vi "Instrument Manager Loop.vi"(8 "System Control":refnum<queue>, 11 "Instrument Manager":refnum<queue>) -> (0 "error out":errorcluster)   [LabVIEW 2020, in "ChromTech Series III Plugin.lvlib" / "Instrument Manager.lvlib"]
uses:
  Instrument Manager/Instrument Manager.lvlib
  support/Message Queue/Message Cluster.ctl
  Instrument Manager/Instrument State.ctl
  <vilib>/Utility/error.llb/Error Cluster From Error Code.vi
  <vilib>/ErrorRing/Error Ring.xnode
  support/Message Queue/Message Queue.lvlib
  ChromTech Series III Plugin.lvlib
  <instrlib>/ChromTech Series III Pump/ChromTech Series III Pump.lvlib
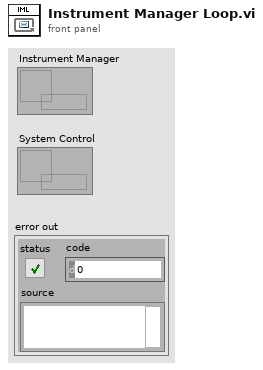
[diagram p1: front panel]
types:
  T1 = typedef "ChromTech Series III Plugin.lvlib/Instrument Manager.lvlib/Instrument State.ctl" = cluster{"VISA Resource":refnum<visa-resource-name>, "Flow Rate":dbl, "Running":bool, "Running Since":timestamp, "Pressure Data Point":cluster{"Time Stamp":timestamp, "Value":dbl}, "Upper Pressure Fault":bool, "Lower Pressure Fault":bool, "Motor Stall Fault":bool, "Sampling Rate (sec/sample)":dbl, "Retry Attempts":i32}
  T2 = cluster{"seconds since 1Jan1904":timestamp, "Pressure":i32}
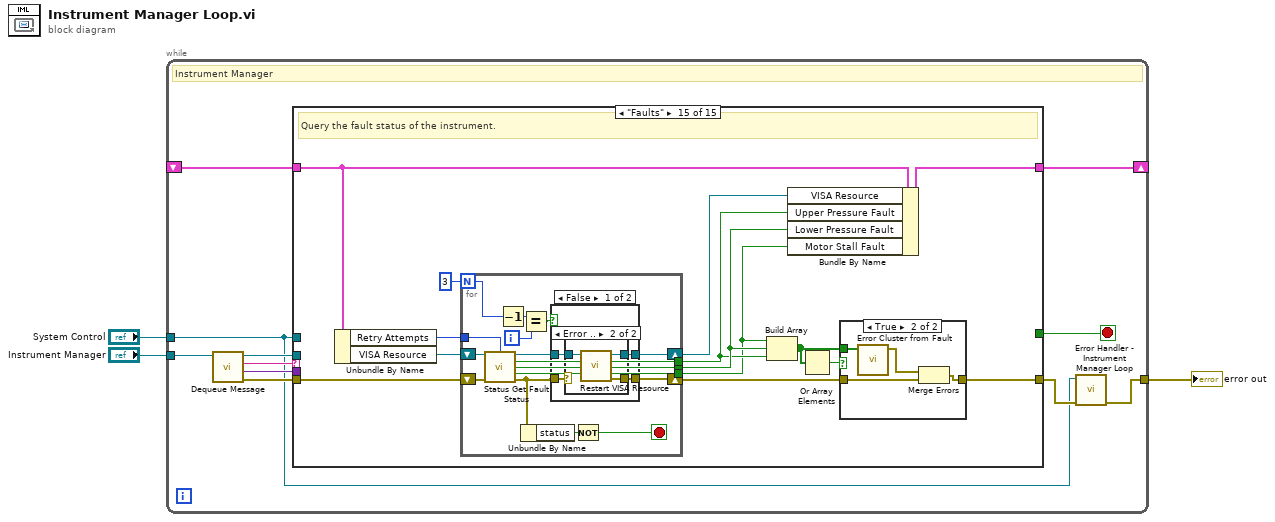
[diagram p0: block diagram]
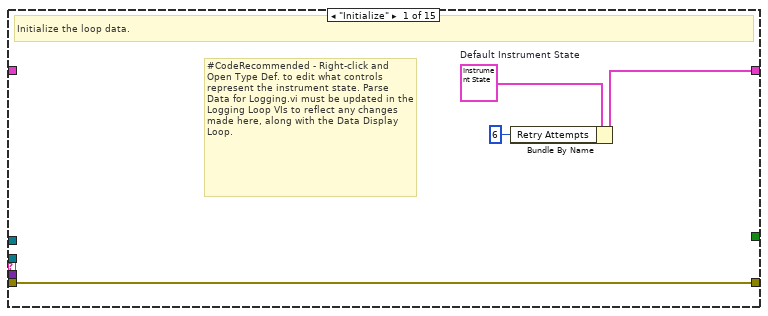
[diagram p2: hidden frame]
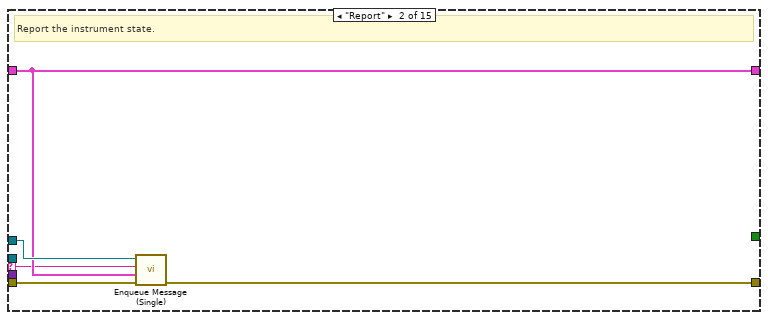
[diagram p3: hidden frame]
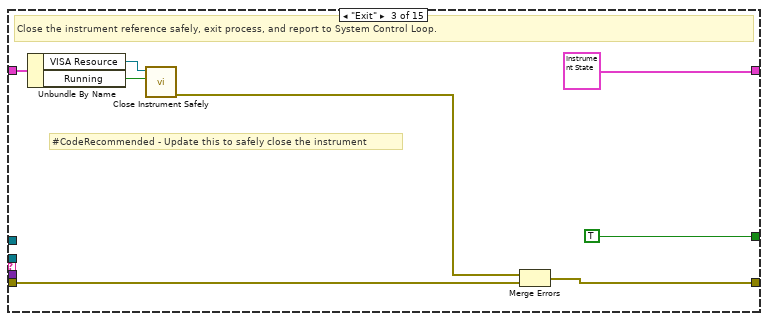
[diagram p4: hidden frame]
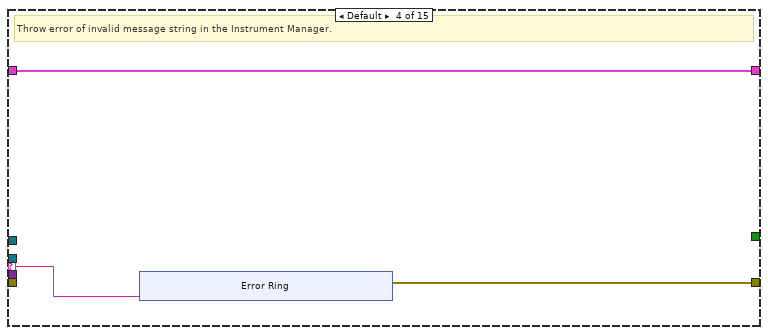
[diagram p5: hidden frame]
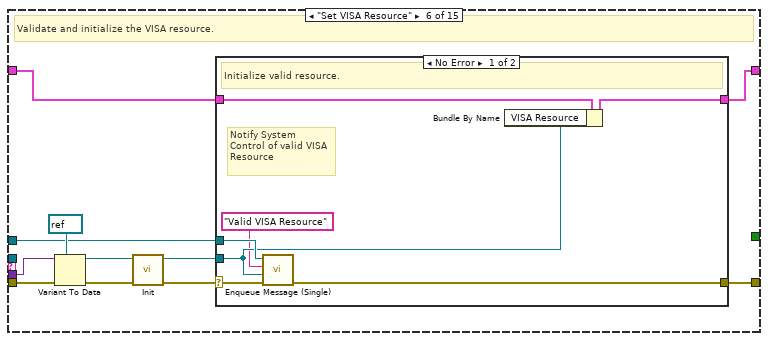
[diagram p7: hidden frame]
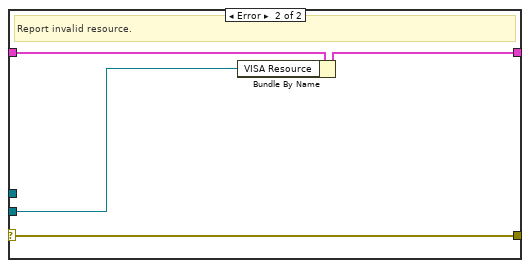
[diagram p8: hidden frame]
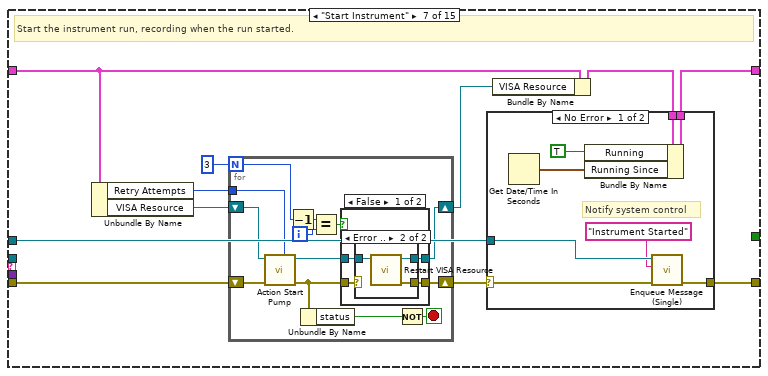
[diagram p9: hidden frame]
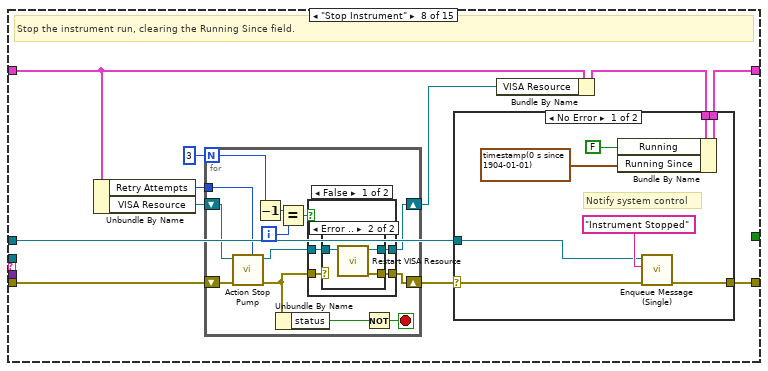
[diagram p13: hidden frame]
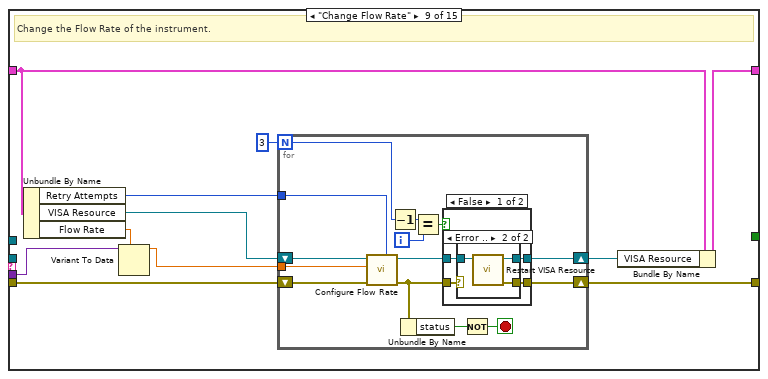
[diagram p17: hidden frame]
diagram:
  n1 = while {
    tunnel: "Instrument Manager" -> [w14]
    tunnel: "System Control" -> [w4]
    tunnel: [w8] -> w1
    shift-right: [w6] -> _
    shift-left: _ -> [w7]
    stop <- w5 stop-if-true
    # "Instrument Manager"
    n2 = call "Dequeue Message.vi"("Message Queue"=w14) -> ("error out"=w10:errorcluster, "Message Data"=w11:variant, "Message"=w13:string, "dup Message Queue"=w12:refnum<queue>)  [unwired: 7 in]
    n3 = case shown="\"Faults\"" w13 {
      selector: w13 -> [_ w19 _ w33 _ _ _ _ _ _ _ _ _ _ _]
      tunnel: w12 -> [_ _ _ _ _ _ _ _ _ _ _ _ _ _ _]
      tunnel: w4 -> [_ w22 _ _ _ w44 w75 w120 _ _ _ _ _ _ _]
      tunnel: w11 -> [_ _ _ _ _ w51 _ _ w166 _ w194 _ _ _ _]
      tunnel: w10 -> [w17 w23 w26 _ w42 w50 w73 w118 w161 w193 w199 w207 w240 w278 w317]
      tunnel: [w17 w21 w25 w32 w42 w54 w76 w121 w160 w193 w199 w206 w239 w276 w310] -> w9
      tunnel: w7 -> [_ w20 w31 w34 w43 w53 w72 w116 w165 w192 w196 w205 w241 w275 w314]
      tunnel: [w16 w20 T1 {"VISA Resource"="", "Flow Rate"=0.0, "Running"=FALSE, "Running Since"=timestamp(0 s since 1904-01-01), "Pressure Data Point"={"Time Stamp"=timestamp(0 s since 1904-01-01), "Value"=0.0}, "Upper Pressure Fault"=FALSE, "Lower Pressure Fault"=FALSE, "Motor Stall Fault"=FALSE, "Sampling Rate (sec/sample)"=0.0, "Retry Attempts"=0} w34 w43 w52 w74 w119 w157 w192 w195 w208 w244 w277 w316] -> w6
      tunnel: [_ _ TRUE _ _ _ _ _ _ _ _ _ _ _ _] -> w5
      frame "Initialize" {
        w18 = T1 {"VISA Resource"="", "Flow Rate"=0.0, "Running"=FALSE, "Running Since"=timestamp(0 s since 1904-01-01), "Pressure Data Point"={"Time Stamp"=timestamp(0 s since 1904-01-01), "Value"=0.0}, "Upper Pressure Fault"=FALSE, "Lower Pressure Fault"=FALSE, "Motor Stall Fault"=FALSE, "Sampling Rate (sec/sample)"=0.0, "Retry Attempts"=0}  # Default Instrument State
        # "#CodeRecommended - Right-click and Open Type Def. to edit what controls represent the instrument state. Parse Data for Logging.vi must be updated in the Logging Loop VIs to reflect any changes made here, along with the Data Display Loop."
        # "Initialize the loop data."
        n4 = Bundle By Name(cluster=w18, "Retry Attempts"=6) -> (w16:T1)
      }
      frame "Report" {
        # "Report the instrument state."
        n5 = call "Enqueue Message (Single).vi"("error in (no error)"=w23, "Message Data"=w20, "Message"=w19, "Message Queue"=w22) -> ("error out"=w21:errorcluster)  [unwired: 6 in, 1 out]
      }
      frame "Exit" {
        # "#CodeRecommended - Update this to safely close the instrument"
        # "Close the instrument reference safely, exit process, and report to System Control Loop."
        n6 = Unbundle By Name(w31) -> ("VISA Resource"=w29:refnum<visa-resource-name>, "Running"=w30:bool)
        n7 = call "Close Instrument Safely.vi"("Running (F)"=w30, "VISA Refnum in"=w29) -> ("error out"=w24:errorcluster)  [unwired: 9 in]
        n8 = Merge Errors(w24, w26) -> (w25:errorcluster)
      }
      frame Default {
        # "Throw error of invalid message string in the Instrument Manager."
        n9 = xnode "Error Ring"("parameter 0"=w33) -> ("error out"=w32:errorcluster)
      }
      frame "--- Copy This Frame ---" {
        # "Copy this frame and add responses to instrument specific messages."
      }
      frame "Set VISA Resource" {
        # "Validate and initialize the VISA resource."
        n10 = Variant To Data(error in=w50, type=refnum<visa-resource-name> refnum, Variant=w51) -> (data=w48:refnum<visa-resource-name>, error out=w49:errorcluster)
        n11 = call "Init.vi"("error in (no error)"=w49, "VISA resource in"=w48) -> ("error out"=w45:errorcluster, "VISA resource out"=w46:refnum<visa-resource-name>)  [unwired: 8 in]
        n12 = case shown="No Error" w45 {
          selector: w45 -> [w60 w62]
          tunnel: w46 -> [w57 w63]
          tunnel: [w59 w62] -> w54
          tunnel: w53 -> [w61 w65]
          tunnel: [w55 w64] -> w52
          tunnel: w44 -> [w58 _]
          frame No Error {
            # "Notify System Control of valid VISA Resource"
            # "Initialize valid resource."
            n13 = call "Enqueue Message (Single).vi"("error in (no error)"=w60, "Message Data"=w57, "Message"="Valid VISA Resource", "Message Queue"=w58) -> ("error out"=w59:errorcluster)  [unwired: 6 in, 1 out]
            n14 = Bundle By Name(cluster=w61, "VISA Resource"=w57) -> (w55:T1)
          }
          frame Error {
            # "Report invalid resource."
            n15 = Bundle By Name(cluster=w65, "VISA Resource"=w63) -> (w64:T1)
          }
        }
      }
      frame "Start Instrument" {
        # "Start the instrument run, recording when the run started."
        n16 = Unbundle By Name(w72) -> ("Retry Attempts"=w69:i32, "VISA Resource"=w71:refnum<visa-resource-name>)
        n17 = for {
          N: 3 -> [w80]
          tunnel: w69 -> [w88]
          shift-right: [w85] -> w70
          shift-left: w73 -> [w82]
          shift-right: [w77] -> w66
          shift-left: w71 -> [w89]
          i -> [w81]
          stop <- w86 stop-if-true
          n18 = call <instrlib>:"Action Start Pump.vi"("Retry Attempts (0)"=w88, "error in"=w82, "VISA resource name"=w89) -> ("error out"=w83:errorcluster, "VISA resource name out"=w84:refnum<visa-resource-name>)  [unwired: 7 in]
          n19 = Decrement(x=w80) -> (x-1=w79:i32)
          n20 = Unbundle By Name(w83) -> ("status"=w87:bool)
          n21 = Equal?(x=w79, y=w81) -> (x = y?=w78:bool)
          n22 = case shown="False" w78 {
            tunnel: [w93 w100] -> w85
            tunnel: w84 -> [w92 w99]
            tunnel: w83 -> [w91 w100]
            tunnel: [w90 w99] -> w77
            frame False {
              n23 = case shown="Error .." w91 {
                selector: w91 -> [w95 _]
                tunnel: [w95 w98] -> w93
                tunnel: w92 -> [w94 w97]
                tunnel: [w94 w96] -> w90
                frame No Error {
                }
                frame Error {
                  n24 = call "Restart VISA Resource.vi"("VISA Refnum in"=w97) -> ("error out"=w98:errorcluster, "VISA resource name out"=w96:refnum<visa-resource-name>)  [unwired: 9 in]
                }
              }
            }
            frame True {
            }
          }
          n25 = Not(x=w87) -> (.not. x?=w86:bool)
        }
        n26 = Bundle By Name(cluster=w72, "VISA Resource"=w66) -> (w67:T1)
        n27 = case shown="No Error" w70 {
          selector: w70 -> [w101 w110]
          tunnel: [w108 w110] -> w76
          tunnel: w75 -> [w107 _]
          tunnel: [w105 w109] -> w74
          tunnel: w67 -> [w102 w109]
          frame No Error {
            # "Notify system control"
            n28 = Get Date/Time In Seconds() -> (seconds since 1Jan1904=w103:timestamp)
            n29 = Bundle By Name(cluster=w102, "Running"=TRUE, "Running Since"=w103) -> (w105:T1)
            n30 = call "Enqueue Message (Single).vi"("error in (no error)"=w101, "Message"="Instrument Started", "Message Queue"=w107) -> ("error out"=w108:errorcluster)  [unwired: 7 in, 1 out]
          }
          frame Error {
          }
        }
      }
      frame "Stop Instrument" {
        # "Stop the instrument run, clearing the Running Since field."
        n31 = Unbundle By Name(w116) -> ("Retry Attempts"=w114:i32, "VISA Resource"=w115:refnum<visa-resource-name>)
        n32 = for {
          N: 3 -> [w124]
          tunnel: w114 -> [w133]
          shift-right: [w126] -> w117
          shift-left: w118 -> [w132]
          shift-right: [w122] -> w111
          shift-left: w115 -> [w134]
          i -> [w123]
          stop <- w130 stop-if-true
          n33 = call <instrlib>:"Action Stop Pump.vi"("Retry Attempts (0)"=w133, "error in"=w132, "VISA resource name"=w134) -> ("error out"=w127:errorcluster, "VISA resource name out"=w125:refnum<visa-resource-name>)  [unwired: 7 in]
          n34 = Decrement(x=w124) -> (x-1=w129:i32)
          n35 = Unbundle By Name(w127) -> ("status"=w131:bool)
          n36 = Equal?(x=w129, y=w123) -> (x = y?=w128:bool)
          n37 = case shown="False" w128 {
            tunnel: [w138 w145] -> w126
            tunnel: w125 -> [w137 w144]
            tunnel: w127 -> [w136 w145]
            tunnel: [w135 w144] -> w122
            frame False {
              n38 = case shown="Error .." w136 {
                selector: w136 -> [w140 _]
                tunnel: [w140 w143] -> w138
                tunnel: w137 -> [w139 w142]
                tunnel: [w139 w141] -> w135
                frame No Error {
                }
                frame Error {
                  n39 = call "Restart VISA Resource.vi"("VISA Refnum in"=w142) -> ("error out"=w143:errorcluster, "VISA resource name out"=w141:refnum<visa-resource-name>)  [unwired: 9 in]
                }
              }
            }
            frame True {
            }
          }
          n40 = Not(x=w131) -> (.not. x?=w130:bool)
        }
        n41 = Bundle By Name(cluster=w116, "VISA Resource"=w111) -> (w112:T1)
        n42 = case shown="No Error" w117 {
          selector: w117 -> [w146 w155]
          tunnel: w112 -> [w153 w154]
          tunnel: [w152 w155] -> w121
          tunnel: w120 -> [w150 _]
          tunnel: [w149 w154] -> w119
          frame No Error {
            # "Notify system control"
            n43 = Bundle By Name(cluster=w153, "Running"=FALSE, "Running Since"=timestamp(0 s since 1904-01-01)) -> (w149:T1)
            n44 = call "Enqueue Message (Single).vi"("error in (no error)"=w146, "Message"="Instrument Stopped", "Message Queue"=w150) -> ("error out"=w152:errorcluster)  [unwired: 7 in, 1 out]
          }
          frame Error {
          }
        }
      }
      frame "Change Flow Rate" {
        # "Change the Flow Rate of the instrument."
        n45 = Unbundle By Name(w165) -> ("Retry Attempts"=w159:i32, "VISA Resource"=w163:refnum<visa-resource-name>, "Flow Rate"=w164:dbl)
        n46 = Variant To Data(type=w164, Variant=w166) -> (data=w162:dbl)  [unwired: 1 in, 1 out]
        n47 = for {
          N: 3 -> [w169]
          tunnel: w162 -> [w179]
          tunnel: w159 -> [w178]
          shift-right: [w171] -> w160
          shift-left: w161 -> [w177]
          shift-right: [w167] -> w156
          shift-left: w163 -> [w180]
          i -> [w168]
          stop <- w175 stop-if-true
          n48 = call <instrlib>:"Configure Flow Rate.vi"("Retry Attempts (0)"=w178, "error in"=w177, "Flow Input (ml/min)"=w179, "VISA resource name"=w180) -> ("error out"=w172:errorcluster, "VISA resource name out"=w170:refnum<visa-resource-name>)  [unwired: 6 in]
          n49 = Decrement(x=w169) -> (x-1=w174:i32)
          n50 = Unbundle By Name(w172) -> ("status"=w176:bool)
          n51 = Equal?(x=w174, y=w168) -> (x = y?=w173:bool)
          n52 = case shown="False" w173 {
            tunnel: [w184 w191] -> w171
            tunnel: w170 -> [w183 w190]
            tunnel: w172 -> [w182 w191]
            tunnel: [w181 w190] -> w167
            frame False {
              n53 = case shown="Error .." w182 {
                selector: w182 -> [w186 _]
                tunnel: [w186 w189] -> w184
                tunnel: w183 -> [w185 w188]
                tunnel: [w185 w187] -> w181
                frame No Error {
                }
                frame Error {
                  n54 = call "Restart VISA Resource.vi"("VISA Refnum in"=w188) -> ("error out"=w189:errorcluster, "VISA resource name out"=w187:refnum<visa-resource-name>)  [unwired: 9 in]
                }
              }
            }
            frame True {
            }
          }
          n55 = Not(x=w176) -> (.not. x?=w175:bool)
        }
        n56 = Bundle By Name(cluster=w165, "VISA Resource"=w156) -> (w157:T1)
      }
      frame "--- Copy for Get State Messages ---" {
        # "#CodeNeeded - Use the Bundle by Name function to bundle the new state value into the Instrument State cluster."
        # "#CodeNeeded - Add instrument driver call to query the instrument state requested"
        # "Duplicate this case for messages cases that will query the instrument state."
      }
      frame "Change Retry Attempts" {
        # "Change the number of Retry Attempts when the instrument fails to respond."
        n57 = Unbundle By Name(w196) -> ("Retry Attempts"=w197:i32)
        n58 = Variant To Data(type=w197, Variant=w194) -> (data=w198:i32)  [unwired: 1 in, 1 out]
        n59 = Bundle By Name(cluster=w196, "Retry Attempts"=w198) -> (w195:T1)
      }
      frame "Run State" {
        # "Query the run state of the instrument."
        n60 = Unbundle By Name(w205) -> ("Retry Attempts"=w202:i32, "VISA Resource"=w204:refnum<visa-resource-name>)
        n61 = for {
          N: 3 -> [w210]
          tunnel: [w221] -> w203
          tunnel: w202 -> [w220]
          shift-right: [w213] -> w206
          shift-left: w207 -> [w219]
          shift-right: [w212] -> w200
          shift-left: w204 -> [w222]
          i -> [w209]
          stop <- w217 stop-if-true
          n62 = call <instrlib>:"Status Run State.vi"("Retry Attempts (0)"=w220, "error in (no error)"=w219, "VISA resource name"=w222) -> ("error out"=w214:errorcluster, "Running?"=w221:bool, "VISA resource name out"=w211:refnum<visa-resource-name>)  [unwired: 6 in]
          n63 = Decrement(x=w210) -> (x-1=w216:i32)
          n64 = Unbundle By Name(w214) -> ("status"=w218:bool)
          n65 = Equal?(x=w216, y=w209) -> (x = y?=w215:bool)
          n66 = case shown="False" w215 {
            tunnel: [w226 w233] -> w213
            tunnel: w211 -> [w225 w232]
            tunnel: w214 -> [w224 w233]
            tunnel: [w223 w232] -> w212
            frame False {
              n67 = case shown="Error .." w224 {
                selector: w224 -> [w228 _]
                tunnel: [w228 w231] -> w226
                tunnel: w225 -> [w227 w230]
                tunnel: [w227 w229] -> w223
                frame No Error {
                }
                frame Error {
                  n68 = call "Restart VISA Resource.vi"("VISA Refnum in"=w230) -> ("error out"=w231:errorcluster, "VISA resource name out"=w229:refnum<visa-resource-name>)  [unwired: 9 in]
                }
              }
            }
            frame True {
            }
          }
          n69 = Not(x=w218) -> (.not. x?=w217:bool)
        }
        n70 = Bundle By Name(cluster=w205, "VISA Resource"=w200, "Running"=w203) -> (w208:T1)
      }
      frame "Pressure" {
        # "Query the pressure value of the instrument."
        n71 = Unbundle By Name(w241) -> ("Retry Attempts"=w236:i32, "VISA Resource"=w238:refnum<visa-resource-name>)
        n72 = for {
          N: 3 -> [w246]
          tunnel: [w257] -> w237
          tunnel: w236 -> [w256]
          shift-right: [w250] -> w239
          shift-left: w240 -> [w247]
          shift-right: [w248] -> w234
          shift-left: w238 -> [w258]
          i -> [w245]
          stop <- w254 stop-if-true
          n73 = call <instrlib>:"Status Get Pressure.vi"("Retry Attempts (0)"=w256, "error in"=w247, "VISA resource name"=w258) -> ("error out"=w251:errorcluster, "Pressure"=w257:i32, "VISA resource name out"=w249:refnum<visa-resource-name>)  [unwired: 6 in]
          n74 = Unbundle By Name(w251) -> ("status"=w255:bool)
          n75 = Decrement(x=w246) -> (x-1=w253:i32)
          n76 = Equal?(x=w253, y=w245) -> (x = y?=w252:bool)
          n77 = case shown="False" w252 {
            tunnel: [w262 w269] -> w250
            tunnel: w249 -> [w261 w268]
            tunnel: w251 -> [w260 w269]
            tunnel: [w259 w268] -> w248
            frame False {
              n78 = case shown="Error .." w260 {
                selector: w260 -> [w264 _]
                tunnel: [w264 w267] -> w262
                tunnel: w261 -> [w263 w266]
                tunnel: [w263 w265] -> w259
                frame No Error {
                }
                frame Error {
                  n79 = call "Restart VISA Resource.vi"("VISA Refnum in"=w266) -> ("error out"=w267:errorcluster, "VISA resource name out"=w265:refnum<visa-resource-name>)  [unwired: 9 in]
                }
              }
            }
            frame True {
            }
          }
          n80 = Not(x=w255) -> (.not. x?=w254:bool)
        }
        n81 = Get Date/Time In Seconds() -> (seconds since 1Jan1904=w243:timestamp)
        n82 = Bundle("seconds since 1Jan1904"=w243, "Pressure"=w237) -> (w242:T2)  [unwired: 1 in]
        n83 = Bundle By Name(cluster=w241, "Pressure Data Point"=w242, "VISA Resource"=w234) -> (w244:T1)
      }
      frame "Flow Rate" {
        # "Query the flow rate of the instrument."
        n84 = Unbundle By Name(w275) -> ("Retry Attempts"=w272:i32, "VISA Resource"=w274:refnum<visa-resource-name>)
        n85 = for {
          N: 3 -> [w281]
          tunnel: [w291] -> w273
          tunnel: w272 -> [w290]
          shift-right: [w284] -> w276
          shift-left: w278 -> [w279]
          shift-right: [w282] -> w270
          shift-left: w274 -> [w292]
          i -> [w280]
          stop <- w288 stop-if-true
          n86 = call <instrlib>:"Status Get Flow Rate.vi"("Retry Attempts (0)"=w290, "error in"=w279, "VISA resource name"=w292) -> ("error out"=w285:errorcluster, "Flow Rate"=w291:dbl, "VISA resource name out"=w283:refnum<visa-resource-name>)  [unwired: 6 in]
          n87 = Unbundle By Name(w285) -> ("status"=w289:bool)
          n88 = Decrement(x=w281) -> (x-1=w287:i32)
          n89 = Equal?(x=w287, y=w280) -> (x = y?=w286:bool)
          n90 = Not(x=w289) -> (.not. x?=w288:bool)
          n91 = case shown="False" w286 {
            tunnel: [w296 w303] -> w284
            tunnel: w283 -> [w295 w302]
            tunnel: w285 -> [w294 w303]
            tunnel: [w293 w302] -> w282
            frame False {
              n92 = case shown="Error .." w294 {
                selector: w294 -> [w298 _]
                tunnel: [w298 w301] -> w296
                tunnel: w295 -> [w297 w300]
                tunnel: [w297 w299] -> w293
                frame No Error {
                }
                frame Error {
                  n93 = call "Restart VISA Resource.vi"("VISA Refnum in"=w300) -> ("error out"=w301:errorcluster, "VISA resource name out"=w299:refnum<visa-resource-name>)  [unwired: 9 in]
                }
              }
            }
            frame True {
            }
          }
        }
        n94 = Bundle By Name(cluster=w275, "VISA Resource"=w270, "Flow Rate"=w273) -> (w277:T1)
      }
      frame "Faults" {
        # "Query the fault status of the instrument."
        n95 = Unbundle By Name(w314) -> ("Retry Attempts"=w306:i32, "VISA Resource"=w313:refnum<visa-resource-name>)
        n96 = for {
          N: 3 -> [w323]
          tunnel: [w332] -> w312
          tunnel: [w331] -> w311
          tunnel: [w330] -> w307
          tunnel: w306 -> [w329]
          shift-right: [w319] -> w315
          shift-left: w317 -> [w326]
          shift-right: [w318] -> w304
          shift-left: w313 -> [w333]
          i -> [w322]
          stop <- w327 stop-if-true
          n97 = call <instrlib>:"Status Get Fault Status.vi"("VISA resource name"=w333, "Retry Attempts (0)"=w329, "error in (no error)"=w326) -> ("VISA resource name out"=w321:refnum<visa-resource-name>, "Upper Pressure Fault"=w331:bool, "Lower Pressure Fault"=w332:bool, "Motor Stall Fault"=w330:bool, "error out"=w320:errorcluster)  [unwired: 8 in]
          n98 = Decrement(x=w323) -> (x-1=w325:i32)
          n99 = Equal?(x=w325, y=w322) -> (x = y?=w324:bool)
          n100 = Unbundle By Name(w320) -> ("status"=w328:bool)
          n101 = case shown="False" w324 {
            tunnel: [w337 w344] -> w319
            tunnel: w321 -> [w336 w343]
            tunnel: w320 -> [w335 w344]
            tunnel: [w334 w343] -> w318
            frame False {
              n102 = case shown="Error .." w335 {
                selector: w335 -> [w339 _]
                tunnel: [w339 w342] -> w337
                tunnel: w336 -> [w338 w341]
                tunnel: [w338 w340] -> w334
                frame No Error {
                }
                frame Error {
                  n103 = call "Restart VISA Resource.vi"("VISA Refnum in"=w341) -> ("error out"=w342:errorcluster, "VISA resource name out"=w340:refnum<visa-resource-name>)  [unwired: 9 in]
                }
              }
            }
            frame True {
            }
          }
          n104 = Not(x=w328) -> (.not. x?=w327:bool)
        }
        n105 = Build Array(w307, w312, w311) -> (w308:bool[])
        n106 = Bundle By Name(cluster=w314, "VISA Resource"=w304, "Upper Pressure Fault"=w311, "Lower Pressure Fault"=w312, "Motor Stall Fault"=w307) -> (w316:T1)
        n107 = Or Array Elements(Boolean array=w308) -> (logical OR=w309:bool)
        n108 = case shown="True" w309 {
          tunnel: w315 -> [w345 w349]
          tunnel: [w345 w348] -> w310
          tunnel: w308 -> [_ w346]
          frame False {
          }
          frame True {
            n109 = call "Error Cluster from Fault.vi"("Fault indicators"=w346) -> ("error out"=w347:errorcluster)  [unwired: 10 in]
            n110 = Merge Errors(w347, w349) -> (w348:errorcluster)
          }
        }
      }
    }
    n111 = call "Error Handler - Instrument Manager Loop.vi"("error in (no error)"=w9, "Message Queue"=w4) -> ("dup error in"=w8:errorcluster)  [unwired: 8 in, 1 out]
  }
  "error out" <- w1
